vi "StepperMotorRotaryEncoderRecorder.vi"() -> ()   [LabVIEW 2013]
uses:
  <vilib>/Utility/error.llb/DialogType.ctl
  <vilib>/DAQmx/read.llb/DAQmx Read (Counter DBL 1Chan 1Samp).vi
  GlobalVariables.vi
  <vilib>/DAQmx/miscellaneous.llb/DAQmx Fill In Error Info.vi
  <vilib>/DAQmx/create/channels.llb/DAQmx Create Channel (CI-Position-Angular Encoder).vi
  <vilib>/DAQmx/configure/timing.llb/DAQmx Timing (Sample Clock).vi
  <vilib>/DAQmx/configure/task.llb/DAQmx Configure Logging (TDMS).vi
  <resource>/objmgr/daqmx.rc
panel:
  in  "Position Offset":dbl format="%#_13g"
  in  "Stop Task":bool=TRUE
  in  "Quit":bool=TRUE
  out "Wall Position":dbl
  in  "Configure Logging and Start Task":bool=TRUE
  in  "Reset":bool=TRUE
  in  "Initialize":bool=TRUE
  out "Recording":bool=TRUE
  out "Wall Position File":string
  out "Convert TDMS":bool=TRUE
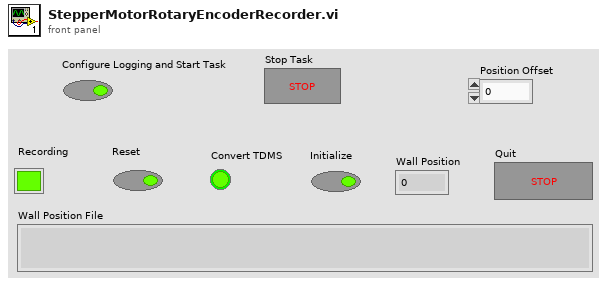
[diagram p1: front panel]
types:
  T1 = typedef "DialogType.ctl" = u16
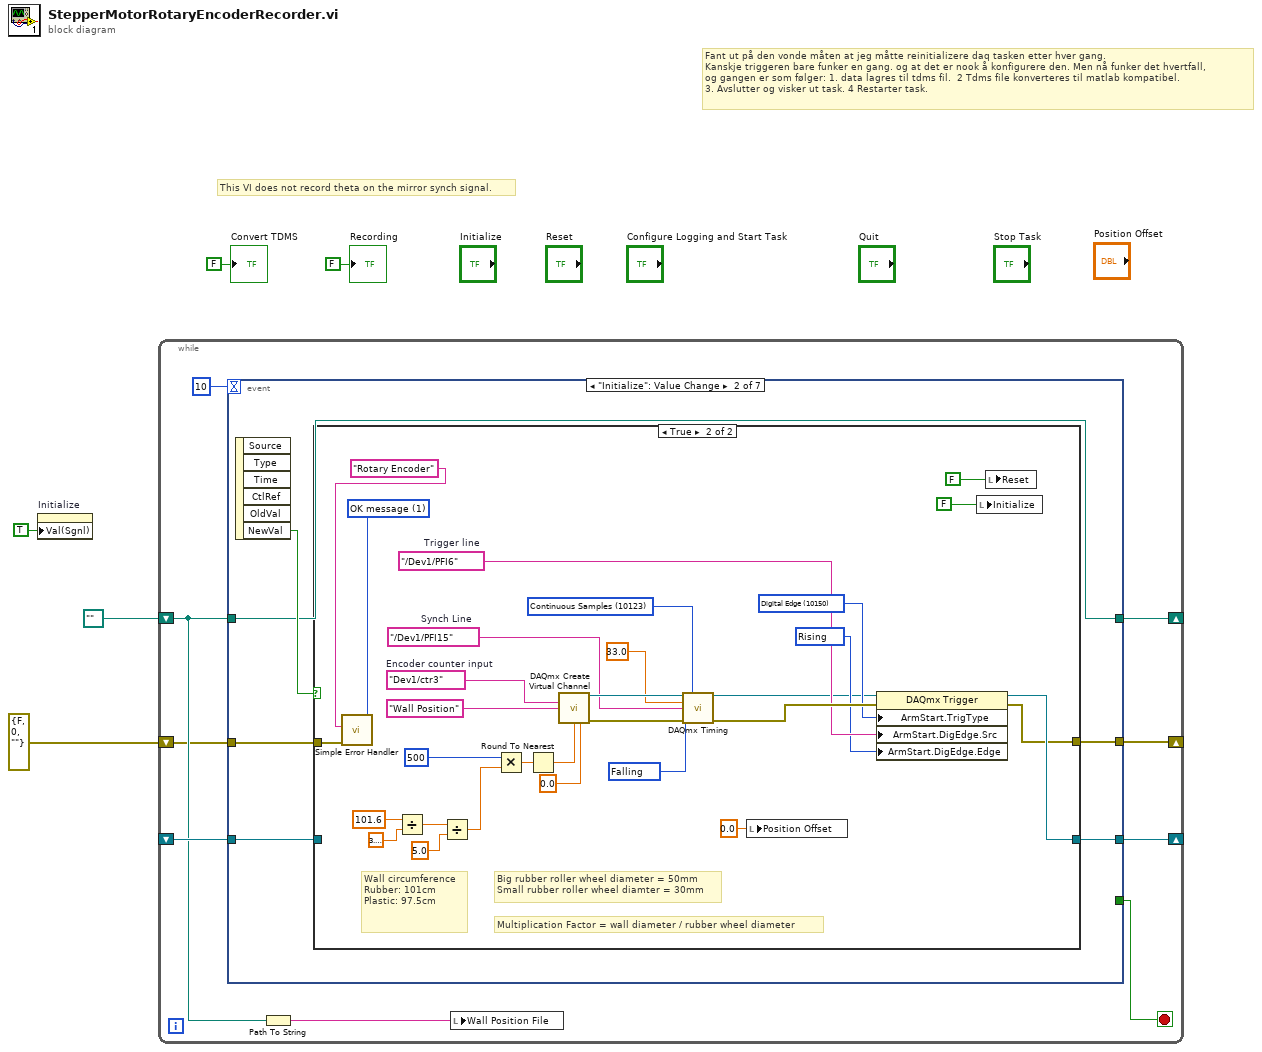
[diagram p0: block diagram]
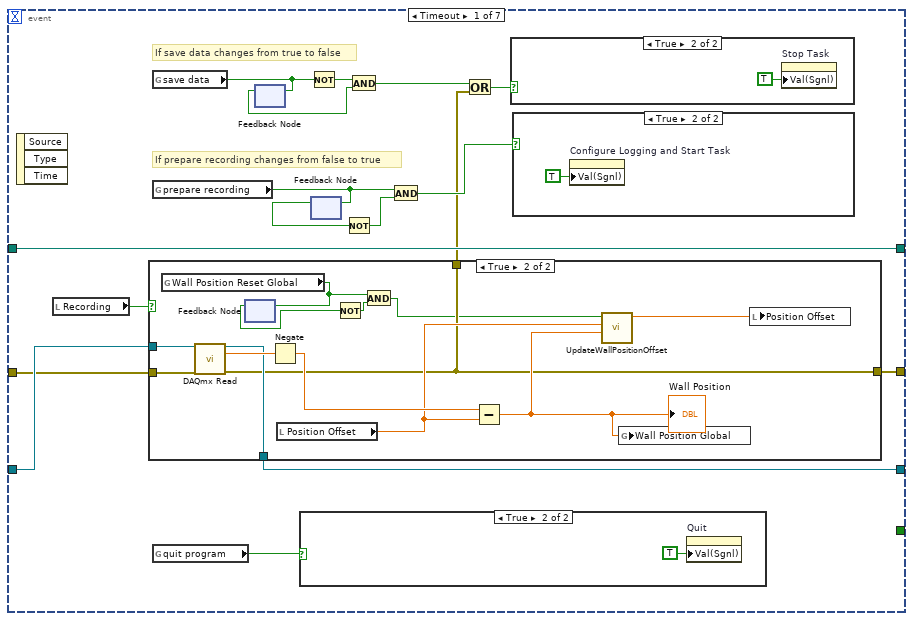
[diagram p2: hidden frame]
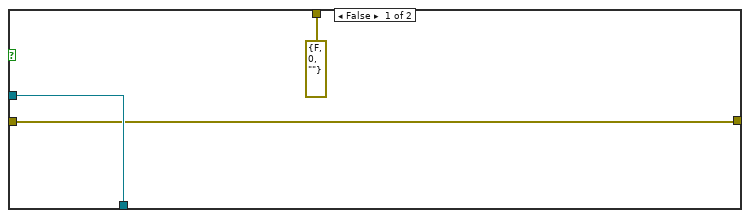
[diagram p6: hidden frame]
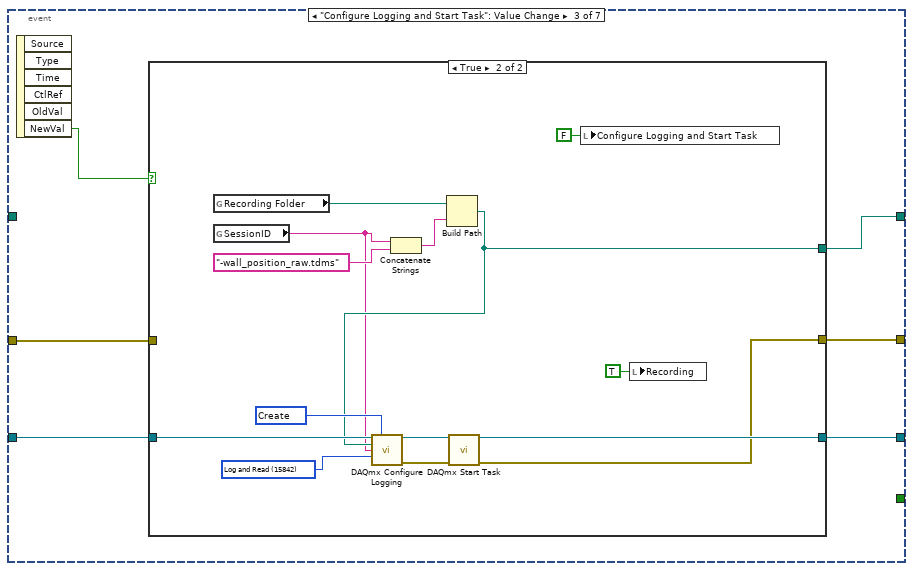
[diagram p8: hidden frame]
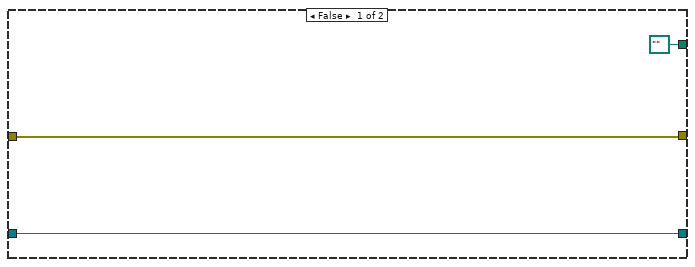
[diagram p9: hidden frame]
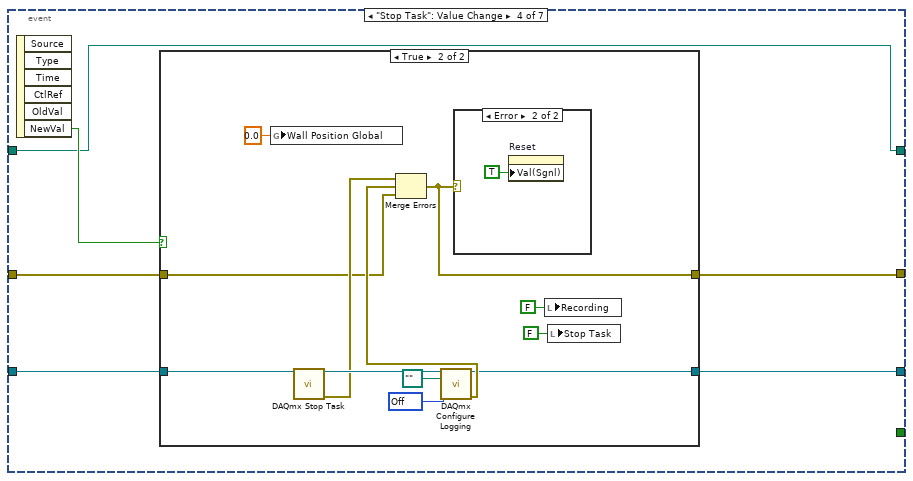
[diagram p10: hidden frame]
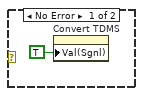
[diagram p12: hidden frame]
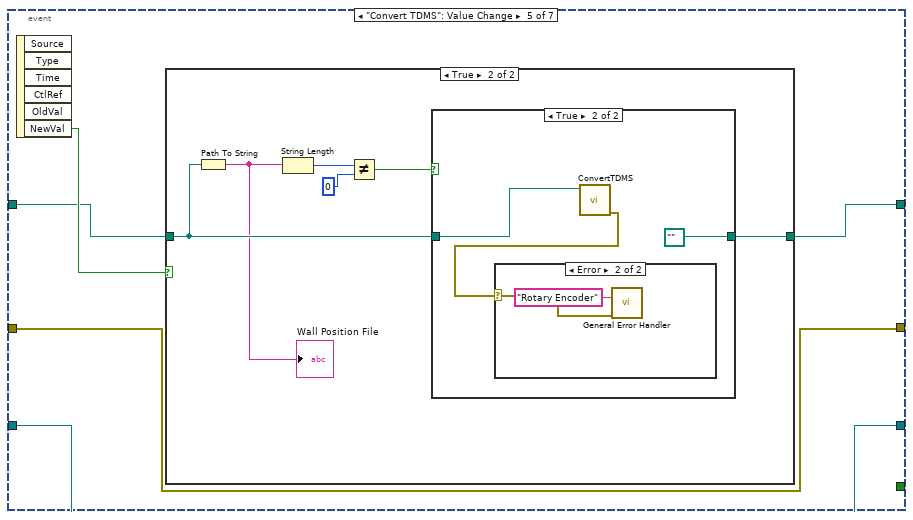
[diagram p13: hidden frame]
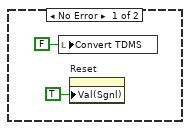
[diagram p16: hidden frame]
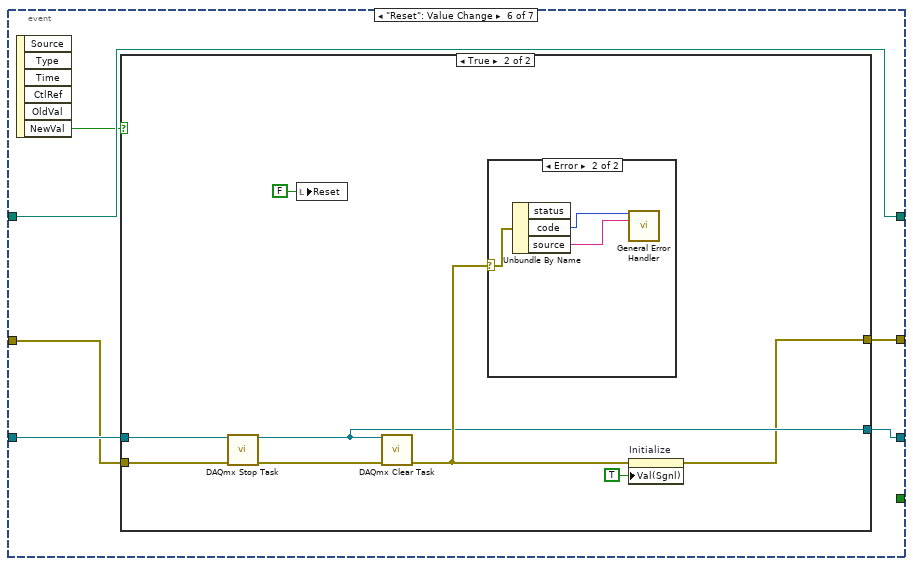
[diagram p17: hidden frame]
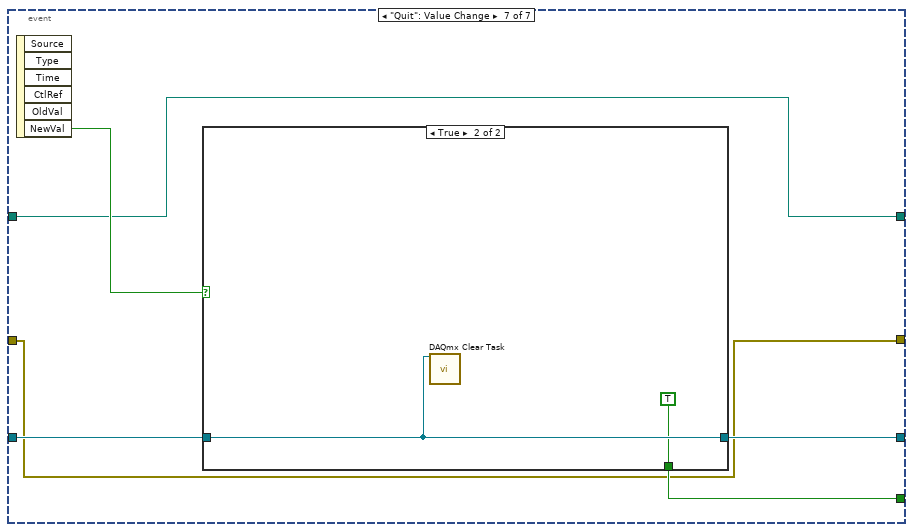
[diagram p20: hidden frame]
diagram:
  # "This VI does not record theta on the mirror synch signal."
  # "Fant ut på den vonde måten at jeg måtte reinitializere daq tasken etter hver gang. \nKanskje triggeren bare funker en gang. og at det er nook å konfigurere den. Men nå funker det hvertfall, \nog gangen er som følger: 1. data lagres til tdms fil.  2 Tdms file konverteres til matlab kompatibel. \n3. Avslutter og visker ut task. 4 Restarter task."
  n1 = property on="Initialize" class="Bool (strict)"("Val(Sgnl)"=TRUE ("Value (Signaling)")) -> ()  [unwired: 2 in, 2 out]
  n2 = while {
    shift-right: [w13] -> _
    shift-left: _ -> [w14]
    shift-right: [w10] -> _
    shift-left: path "" -> [w11]
    shift-right: [w7] -> _
    shift-left: errorcluster {"status"=FALSE, "code"=0, "source"=""} ("error out") -> [w6]
    stop <- w8 stop-if-true
    n3 = event shown="[1] \"Initialize\": Value Change" {
      selector: _ -> [_ _ _ _ _ _ _]
      dyn-events: _ -> [_ _ _ _ _ _ _]
      timeout: 10 -> [_ _ _ _ _ _ _]
      tunnel: [_ _ _ _ _ _ w174] -> w8
      tunnel: w14 -> [w21 w54 w94 w117 w137 w157 w178]
      tunnel: [w20 w55 w93 w116 w137 w156 w177] -> w13
      tunnel: w11 -> [w31 w53 _ w114 w136 w159 w175]
      tunnel: [w31 w53 w92 w114 w135 w159 w175] -> w10
      tunnel: [w16 w52 w90 w112 w134 w154 w173] -> w7
      tunnel: w6 -> [w15 w51 w89 w113 w134 w155 w173]
      event Timeout {
        # "If prepare recording changes from false to true"
        # "If save data changes from true to false"
        n4 = event-data() -> ()  [unwired: 1 in, 3 out]
        n5 = local read "Recording"() -> (w30:bool)
        n6 = case shown="True" w30 {
          tunnel: w21 -> [w37 w50]
          tunnel: [w37 w48] -> w20
          tunnel: [errorcluster {"status"=FALSE, "code"=0, "source"=""} ("error out") w40] -> w18
          tunnel: [w35 w40] -> w16
          tunnel: w15 -> [w35 w39]
          frame False {
          }
          frame True {
            n7 = global read "GlobalVariables.vi" "Wall Position Reset Global"() -> (w44:bool)
            n8 = call-poly <vilib>:"DAQmx Read.vi"("task/channels in"=w50, "error in"=w39) -> ("task out"=w48:refnum<k21>, "data"=w49:dbl, "error out"=w40:errorcluster)  [unwired: 11 in]
            n9 = feedback-in #1(w44) -> ()
            n10 = feedback #1() -> (w42:bool)  [unwired: 1 in]
            n11 = Negate(x=w49) -> (-x=w47:dbl)
            n12 = local read "Position Offset"() -> (w46:dbl)
            n13 = Not(x=w42) -> (.not. x?=w43:bool)
            n14 = And(x=w44, y=w43) -> (x .and. y?=w38:bool)
            n15 = Subtract(x=w47, y=w46) -> (x-y=w45:dbl)
            "Wall Position" <- w45
            n16 = call "UpdateWallPositionOffset.vi"("Sampled Position"=w45, "Wall Position Offset In"=w46, "Ref Switch"=w38) -> ("Wall Position Offset Out"=w41:dbl)  [unwired: 8 in]
            n17 = global write "GlobalVariables.vi" "Wall Position Global"(w45) -> ()
            n18 = local write "Position Offset"(w41) -> ()
          }
        }
        n19 = global read "GlobalVariables.vi" "save data"() -> (w28:bool)
        n20 = global read "GlobalVariables.vi" "prepare recording"() -> (w26:bool)
        n21 = global read "GlobalVariables.vi" "quit program"() -> (w22:bool)
        n22 = feedback #2() -> (w27:bool)  [unwired: 1 in]
        n23 = feedback-in #2(w28) -> ()
        n24 = case shown="True" w22 {
          frame False {
          }
          frame True {
            n25 = property on="Quit" class="Bool (strict)"("Val(Sgnl)"=TRUE ("Value (Signaling)")) -> ()  [unwired: 2 in, 2 out]
          }
        }
        n26 = Not(x=w28) -> (.not. x?=w29:bool)
        n27 = feedback #3() -> (w24:bool)  [unwired: 1 in]
        n28 = feedback-in #3(w26) -> ()
        n29 = Not(x=w24) -> (.not. x?=w25:bool)
        n30 = And(x=w29, y=w27) -> (x .and. y?=w19:bool)
        n31 = And(x=w26, y=w25) -> (x .and. y?=w23:bool)
        n32 = Or(x=w19, y=w18) -> (x .or. y?=w17:bool)
        n33 = case shown="True" w17 {
          frame False {
          }
          frame True {
            n34 = property on="Stop Task" class="Bool (strict)"("Val(Sgnl)"=TRUE ("Value (Signaling)")) -> ()  [unwired: 2 in, 2 out]
          }
        }
        n35 = case shown="True" w23 {
          frame False {
          }
          frame True {
            n36 = property on="Configure Logging and Start Task" class="Bool (strict)"("Val(Sgnl)"=TRUE ("Value (Signaling)")) -> ()  [unwired: 2 in, 2 out]
          }
        }
      }
      event "Initialize": Value Change {
        n37 = event-data() -> ("NewVal"=w56:bool)  [unwired: 1 in, 5 out]
        n38 = case shown="True" w56 {
          tunnel: [w58 w72] -> w55
          tunnel: w54 -> [w58 _]
          tunnel: [w57 w62] -> w52
          tunnel: w51 -> [w57 w61]
          frame False {
          }
          frame True {
            w60 = T1 1 items=["no dialog", "OK message", "continue or stop message", "OK message + warnings", "continue/stop + warnings"] ("type of dialog (OK msg:1)")
            w74 = 10150 items=["Digital Edge"=10150, "None"=10230] ("ArmStart.TrigType")
            w75 = 10280 items=["Rising"=10280, "Falling"=10171] ("ArmStart.DigEdge.Edge")
            w77 = tag "/Dev1/PFI6"  # Trigger line
            w88 = 10171 items=["Rising"=10280, "Falling"=10171] ("active edge")
            w85 = 10123 items=["Finite Samples"=10178, "Continuous Samples"=10123, "Hardware Timed Single Point"=12522] ("sample mode")
            w76 = tag "/Dev1/PFI15"  # Synch Line
            w84 = tag "Dev1/ctr3"  # Encoder counter input
            # "Multiplication Factor = wall diameter / rubber wheel diameter"
            # "Big rubber roller wheel diameter = 50mm\nSmall rubber roller wheel diamter = 30mm"
            # "Wall circumference\nRubber: 101cm\nPlastic: 97.5cm"
            n39 = call <vilib>:"Simple Error Handler.vi"("error source (\" \")"="Rotary Encoder" ("[error source] (\" \")"), "type of dialog (OK msg:1)"=w60, "error in (no error)"=w61) -> ()  [unwired: 2 in, 5 out]
            n40 = Divide(x=101.6, y=3.141592653589793) -> (x/y=w65:dbl)
            n41 = Divide(x=w65, y=5.0) -> (x/y=w63:dbl)
            n42 = Multiply(x=u32 500 ("pulses per revolution"), y=w63) -> (x*y=w71:dbl)
            n43 = Round To Nearest(number=w71) -> (nearest integer value=w69:dbl)
            n44 = call-poly <vilib>:"DAQmx Create Virtual Channel.vi"("counter"=w84, "name to assign"="Wall Position", "pulses per revolution"=w69, "initial angle"=0.0) -> ("task out"=w83:refnum<k21>, "error out"=w86:errorcluster)  [unwired: 10 in]
            n45 = call-poly <vilib>:"DAQmx Timing.vi"("task/channels in"=w83, "sample mode"=w85, "rate"=33.0, "source"=w76, "active edge"=w88, "error in"=w86) -> ("task out"=w73:refnum<k21>, "error out"=w87:errorcluster)  [unwired: 8 in]
            n46 = local write "Position Offset"(0.0 ("Position Offset")) -> ()
            n47 = property class="DAQmx Trigger"(reference=w73, error in=w87, "ArmStart.TrigType"=w74, "ArmStart.DigEdge.Src"=w77, "ArmStart.DigEdge.Edge"=w75) -> (reference out=w72:refnum<k21>, error out=w62:errorcluster)
            n48 = local write "Initialize"(FALSE ("Initialize")) -> ()
            n49 = local write "Reset"(FALSE ("Reset")) -> ()
          }
        }
      }
      event "Configure Logging and Start Task": Value Change {
        n50 = event-data() -> ("NewVal"=w91:bool)  [unwired: 1 in, 5 out]
        n51 = case shown="True" w91 {
          tunnel: w94 -> [w97 w109]
          tunnel: [w97 w107] -> w93
          tunnel: [path "" ("appended path") w104] -> w92
          tunnel: [w95 w98] -> w90
          tunnel: w89 -> [w95 _]
          frame False {
          }
          frame True {
            w111 = 15848 items=["Open"=10437, "Open or Create"=15846, "Create or Replace"=15847, "Create"=15848] ("operation")
            w110 = 15842 items=["Off"=10231, "Log"=15844, "Log and Read"=15842] ("logging mode")
            n52 = global read "GlobalVariables.vi" "Recording Folder"() -> (w100:path)
            n53 = global read "GlobalVariables.vi" "SessionID"() -> (w103:string)
            n54 = Concatenate Strings(w103, "-wall_position_raw.tdms" ("string")) -> (w105:string)
            n55 = Build Path(base path=w100, name or relative path=w105) -> (appended path=w104:path)
            n56 = call-poly <vilib>:"DAQmx Configure Logging.vi"("task/channels in"=w109, "operation"=w111, "file path"=w104, "group name"=w103, "logging mode"=w110) -> ("task out"=w108:refnum<k21>, "error out"=w99:errorcluster)  [unwired: 9 in]
            n57 = call <vilib>:"DAQmx Start Task.vi"("task/channels in"=w108, "error in"=w99) -> ("task out"=w107:refnum<k21>, "error out"=w98:errorcluster)  [unwired: 12 in]
            n58 = local write "Configure Logging and Start Task"(FALSE ("Configure Logging and Start Task")) -> ()
            n59 = local write "Recording"(TRUE ("Recording")) -> ()
          }
        }
      }
      event "Stop Task": Value Change {
        n60 = event-data() -> ("NewVal"=w115:bool)  [unwired: 1 in, 5 out]
        n61 = case shown="True" w115 {
          tunnel: w117 -> [w119 w126]
          tunnel: [w119 w125] -> w116
          tunnel: w113 -> [w118 w121]
          tunnel: [w118 w120] -> w112
          frame False {
          }
          frame True {
            w131 = 10231 items=["Off"=10231, "Log"=15844, "Log and Read"=15842] ("logging mode")
            n62 = global write "GlobalVariables.vi" "Wall Position Global"(0.0 ("Wall Position Global")) -> ()
            n63 = call <vilib>:"DAQmx Stop Task.vi"("task/channels in"=w126) -> ("task out"=w129:refnum<k21>, "error out"=w128:errorcluster)  [unwired: 13 in]
            n64 = call-poly <vilib>:"DAQmx Configure Logging.vi"("task/channels in"=w129, "file path"=path "", "logging mode"=w131) -> ("task out"=w125:refnum<k21>, "error out"=w127:errorcluster)  [unwired: 11 in]
            n65 = Merge Errors(w128, w127, w121) -> (w120:errorcluster)
            n66 = case shown="Error" w120 {
              frame No Error {
                n67 = property on="Convert TDMS" class="Bool (strict)"("Val(Sgnl)"=TRUE ("Value (Signaling)")) -> ()  [unwired: 2 in, 2 out]
              }
              frame Error {
                n68 = property on="Reset" class="Bool (strict)"("Val(Sgnl)"=TRUE ("Value (Signaling)")) -> ()  [unwired: 2 in, 2 out]
              }
            }
            n69 = local write "Recording"(FALSE ("Recording")) -> ()
            n70 = local write "Stop Task"(FALSE ("Stop Task")) -> ()
          }
        }
      }
      event "Convert TDMS": Value Change {
        n71 = event-data() -> ("NewVal"=w138:bool)  [unwired: 1 in, 5 out]
        n72 = case shown="True" w138 {
          tunnel: w136 -> [w139 w144]
          tunnel: [w139 w145] -> w135
          frame False {
          }
          frame True {
            n73 = Path To String(path=w144) -> (string=w141:string)
            "Wall Position File" <- w141
            n74 = String Length(string=w141) -> (length=w143:i32)
            n75 = Not Equal?(x=w143, y=0) -> (x != y?=w140:bool)
            n76 = case shown="True" w140 {
              tunnel: w144 -> [w146 w149]
              tunnel: [w146 path ""] -> w145
              frame False {
              }
              frame True {
                n77 = call "ConvertTDMS.vi"("File With RawDaq"=w149) -> ("error"=w147:errorcluster)  [unwired: 10 in]
                n78 = case shown="Error" w147 {
                  selector: w147 -> [_ w153]
                  frame No Error {
                    n79 = local write "Convert TDMS"(FALSE ("Convert TDMS")) -> ()
                    n80 = property on="Reset" class="Bool (strict)"("Val(Sgnl)"=TRUE ("Value (Signaling)")) -> ()  [unwired: 2 in, 2 out]
                  }
                  frame Error {
                    n81 = call <vilib>:"General Error Handler.vi"("[error source] (\" \")"="Rotary Encoder" ("[error source] (\" \")"), "error in (no error)"=w153) -> ()  [unwired: 9 in, 5 out]
                  }
                }
              }
            }
          }
        }
      }
      event "Reset": Value Change {
        n82 = event-data() -> ("NewVal"=w158:bool)  [unwired: 1 in, 5 out]
        n83 = case shown="True" w158 {
          tunnel: w157 -> [w161 w169]
          tunnel: [w161 w164] -> w156
          tunnel: w155 -> [w160 w163]
          tunnel: [w160 w162] -> w154
          frame False {
          }
          frame True {
            n84 = call <vilib>:"DAQmx Stop Task.vi"("task/channels in"=w169, "error in"=w163) -> ("task out"=w164:refnum<k21>, "error out"=w168:errorcluster)  [unwired: 12 in]
            n85 = local write "Reset"(FALSE ("Reset")) -> ()
            n86 = call <vilib>:"DAQmx Clear Task.vi"("task in"=w164, "error in"=w168) -> ("error out"=w165:errorcluster)  [unwired: 13 in]
            n87 = case shown="Error" w165 {
              selector: w165 -> [_ w170]
              frame No Error {
              }
              frame Error {
                n88 = Unbundle By Name(w170) -> ("code"=w172:i32, "source"=w171:string)  [unwired: 1 out]
                n89 = call <vilib>:"General Error Handler.vi"("[error code] (0)"=w172, "[error source] (\" \")"=w171) -> ()  [unwired: 9 in, 5 out]
              }
            }
            n90 = property on="Initialize" class="Bool (strict)"(error in=w165, "Val(Sgnl)"=TRUE ("Value (Signaling)")) -> (error out=w162:errorcluster)  [unwired: 1 in, 1 out]
          }
        }
      }
      event "Quit": Value Change {
        n91 = event-data() -> ("NewVal"=w176:bool)  [unwired: 1 in, 5 out]
        n92 = case shown="True" w176 {
          tunnel: w178 -> [w180 w182]
          tunnel: [w180 w182] -> w177
          tunnel: [FALSE TRUE] -> w174
          frame False {
          }
          frame True {
            n93 = call <vilib>:"DAQmx Clear Task.vi"("task in"=w182) -> ()  [unwired: 14 in, 1 out]
          }
        }
      }
    }
    n94 = Path To String(path=w11) -> (string=w12:string)
    n95 = local write "Wall Position File"(w12) -> ()
  }
  "Convert TDMS" <- FALSE ("Convert TDMS")
  "Recording" <- FALSE ("Recording")
